vi "Distributor - STOP - Child Actors.vi"(8 "error in (no error)":errorcluster, 11 "Parent_Class in":refnum<class "Message_Distributor_Class.lvclass">) -> (0 "error out":errorcluster, 3 "Parent_Class out":refnum<class "Message_Distributor_Class.lvclass">)   [LabVIEW 2023, in "Actor_Message_Distributor.lvlib" / "Message_Distributor_Class.lvclass"]
uses:
  Message_Distributor_Class.lvclass
  Message_Distributor_Class.lvclass/Message_Distributor_Class.ctl
  <vilib>/ActorFramework/Message Enqueuer/Message Enqueuer.lvclass/Message Enqueuer.ctl
  <vilib>/ActorFramework/Message Enqueuer/Enqueue.vi
  <vilib>/ActorFramework/Stop Msg/Stop Msg.lvclass
  Applications/National Instruments/LabVIEW 2023 64-bit/vi.lib/ActorFramework/Message/Message.lvclass
  <vilib>/ActorFramework/Message Priority Queue/Priority Enqueue.vi
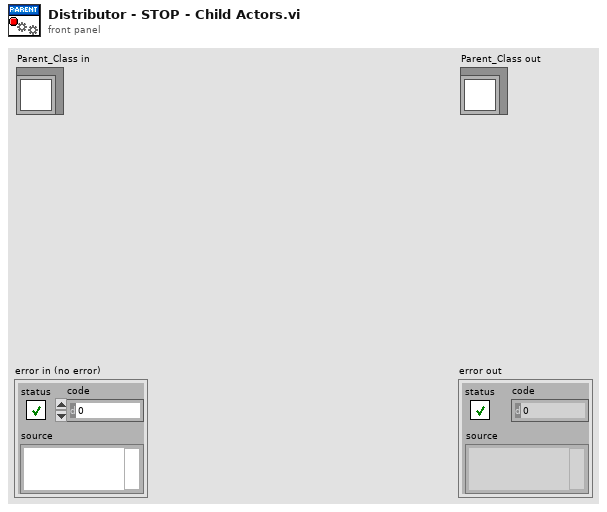
[diagram p1: front panel]
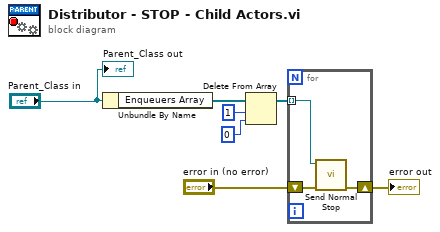
[diagram p0: block diagram]
diagram:
  n1 = Unbundle By Name("Parent_Class in") -> ("Enqueuers Array"=w6:refnum<class "Message Enqueuer.lvclass">[])
  n2 = Delete From Array(array=w6, length=1, index=0) -> (array with subset deleted=w3:refnum<class "Message Enqueuer.lvclass">[])  [unwired: 1 out]
  n3 = for {
    tunnel: w3 -> [w10] mode=indexing
    shift-right: [w8] -> w1
    shift-left: "error in (no error)" -> [w9]
    n4 = call <vilib>:"Send Normal Stop.vi"("error in (no error)"=w9, "Message Enqueuer"=w10) -> ("error out"=w8:errorcluster)  [unwired: 9 in]
  }
  "error out" <- w1
  "Parent_Class out" <- "Parent_Class in"
